vi "elapsedTimePlotWaveformChart.vi"() -> ()   [LabVIEW 2017]
panel:
  out "Elapsed time <s>":dbl format="%#_13g"
  in  "PWM Command":dbl min=0.0 max=255.0 step=1.0
  out "Voltage Chart":waveform(dbl)(graph)
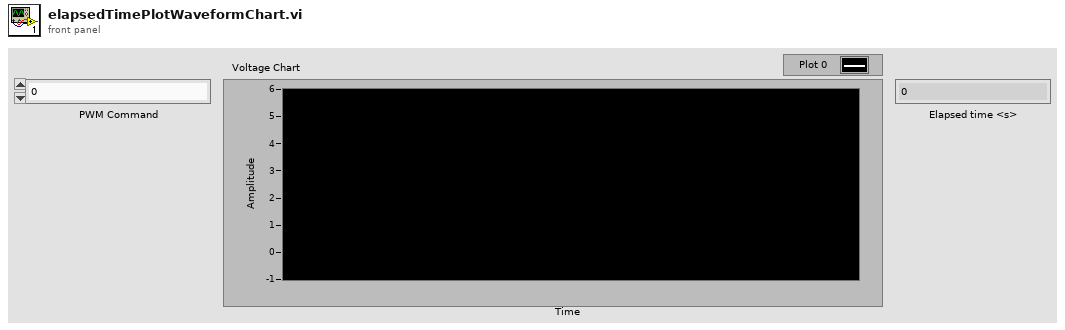
[diagram p1: front panel]
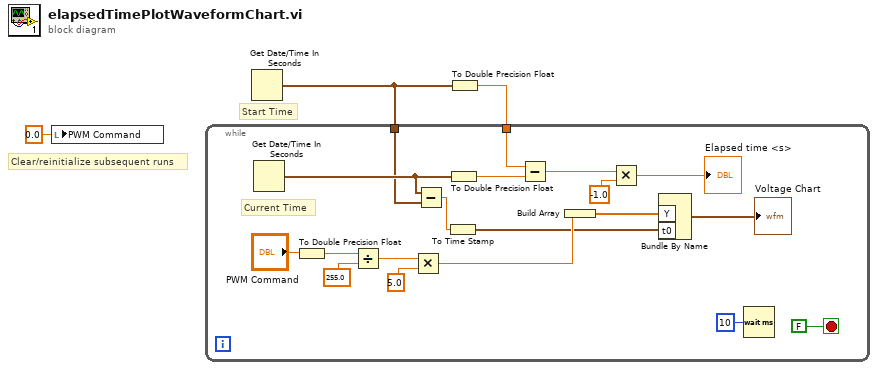
[diagram p0: block diagram]
diagram:
  # "Clear/reinitialize subsequent runs"
  # "Start Time"
  n1 = local write "PWM Command"(0.0 ("PWM Command")) -> ()
  n2 = Get Date/Time In Seconds() -> (seconds since 1Jan1904=w1:timestamp)
  n3 = To Double Precision Float(number=w1) -> (double precision float=w2:dbl)
  n4 = while {
    tunnel: w2 -> [w16]
    tunnel: w1 -> [w6]
    stop <- FALSE stop-if-true
    # "Current Time"
    n5 = Get Date/Time In Seconds() -> (seconds since 1Jan1904=w7:timestamp)
    n6 = To Double Precision Float(number="PWM Command") -> (double precision float=w17:dbl)
    n7 = Divide(x=w17, y=255.0) -> (x/y=w20:dbl)
    n8 = Multiply(x=w20, y=5.0) -> (x*y=w10:dbl)
    n9 = Subtract(x=w7, y=w6) -> (x-y=w5:dbl)
    n10 = To Time Stamp(1:w5) -> (0:w4:timestamp)
    n11 = To Double Precision Float(number=w7) -> (double precision float=w11:dbl)
    n12 = Subtract(x=w16, y=w11) -> (x-y=w15:dbl)
    n13 = Build Array(w10) -> (w9:dbl[])
    n14 = Multiply(x=w15, y=-1.0) -> (x*y=→"Elapsed time <s>":dbl)
    n15 = Bundle By Name("Y"=w9, "t0"=w4) -> (→"Voltage Chart":waveform(dbl))  [unwired: 1 in]
    n16 = Wait (ms)(milliseconds to wait=u32 10) -> ()  [unwired: 1 out]
  }
